vi "Generate Sync Cmd Event.vi"(4 "Task ID":string, 5 "Wait (F)":bool, 6 "Timeout (ms)":u32, 7 "AdHoc Cmd (\"\")":string, 8 "error in (no error)":errorcluster, 9 "vData":variant, 10 "AsyncCmd":T1, 11 "DLP2 in":refnum<class "DLP2.lvclass">) -> (0 "error out":errorcluster, 2 "Return Value":variant, 3 "DLP2 out":refnum<class "DLP2.lvclass">)   [LabVIEW 2022 SP3, in "DLP2.lvclass"]
doc: "Developed by Kevin Thompson\nkevin@thompsonengineering.net\n\nCopyright 2018\nThompson Engineering, LLC"
uses:
  DLP2.lvclass
  DataTypes/AsynCmd_Temp01--enum.ctl
  Common/Controls/TD Sync API Event Data.ctl
  Common/Controls/APIReturnCluster--Cluster.ctl
  Common/Controls/TD Sync API Task State.ctl
  Common/Controls/TD Async CmdMsg EventData--cluster.ctl
  DLP2.lvclass/DLP2.ctl
  Accessors/Get PublicEvents.vi
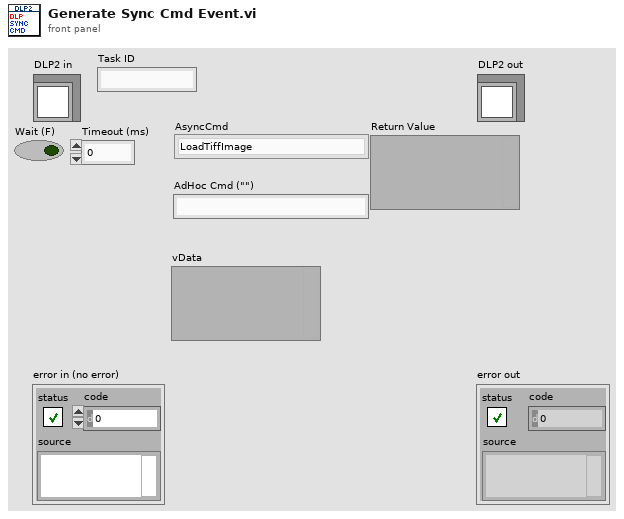
[diagram p1: front panel]
types:
  T1 = typedef "DLP2.lvclass/AsynCmd_Temp01--enum.ctl" = enum16{"LoadTiffImage"}
  T2 = typedef "TD Sync API Task State.ctl" = enum16{"Completed", "Executing", "Errored", "Pending"}
  T3 = typedef "TD Async CmdMsg EventData--cluster.ctl" = cluster{"Time Stamp":timestamp, "CmdMsg":string, "vData":variant}
  T4 = typedef "TD Sync API Event Data.ctl" = cluster{"Task":T5, "Command":variant, "Return Value":variant}
  T5 = typedef "APIReturnCluster--Cluster.ctl" = cluster{"Time Stamp":timestamp, "Timeout (ms)":u32, "Task State":T2, "Task Error":errorcluster, "Task ID":string, "Type":enum16{"API", "CMD"}}
  T6 = typedef "DLP2.lvclass/Public Events--cluster.ctl" = cluster{"Temp01.AsyncCmd Event":refnum<user-event>, "Temp01.AsyncMsg Event":refnum<user-event>, "stop process":refnum<user-event>, "API Incoming Event":refnum<user-event>, "API Executed Event":refnum<user-event>, "API Return Event":refnum<user-event>}
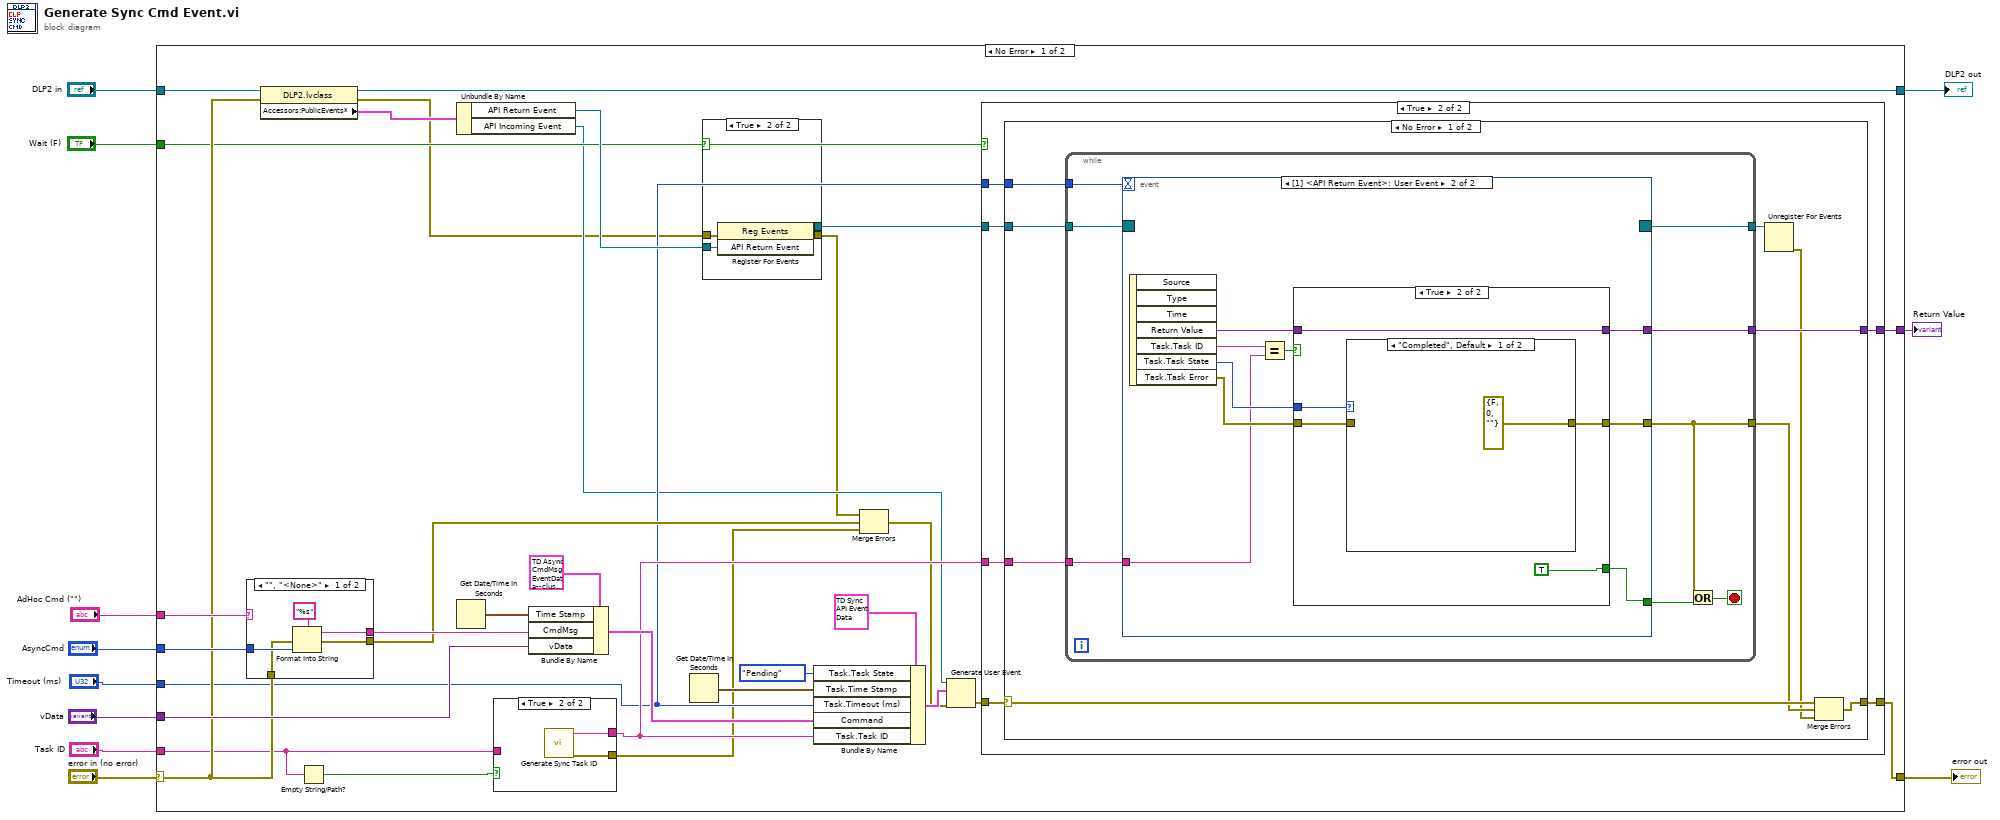
[diagram p0: block diagram]
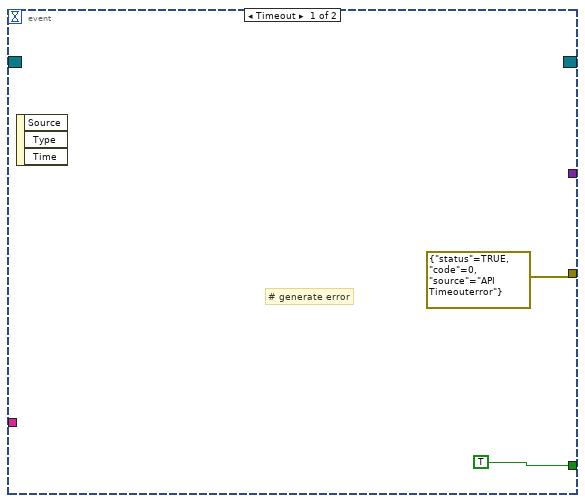
[diagram p3: hidden frame]
diagram:
  n1 = case shown="No Error" "error in (no error)" {
    selector: "error in (no error)" -> [w33 w102]
    tunnel: [w18 w102] -> w10
    tunnel: [w35 w101] -> w8
    tunnel: "DLP2 in" -> [w39 w101]
    tunnel: "AsyncCmd" -> [w37 _]
    tunnel: "vData" -> [w40 _]
    tunnel: "AdHoc Cmd (\"\")" -> [w36 _]
    tunnel: "Wait (F)" -> [w19 _]
    tunnel: "Task ID" -> [w28 _]
    tunnel: "Timeout (ms)" -> [w21 _]
    tunnel: [w17 _] -> w1
    frame No Error {
      n2 = case shown="\"\", \"<None>\"" w36 {
        selector: w36 -> [_ w99]
        tunnel: w37 -> [w97 _]
        tunnel: [w96 w99] -> w41
        tunnel: w33 -> [w95 w100]
        tunnel: [w94 w100] -> w38
        frame "", "<None>" {
          n3 = Format Into String(format string="%s", error in=w95, w97) -> (resulting string=w96:string, error out=w94:errorcluster)  [unwired: 1 in]
        }
        frame Default {
        }
      }
      n4 = property class="DLP2.lvclass"(reference=w39, error in=w33) -> (reference out=w35:refnum<class "DLP2.lvclass">, error out=w13:errorcluster, "Accessors:PublicEvents*"=w34:T6)
      n5 = Empty String/Path?(string/path=w28) -> (empty?=w27:bool)
      n6 = Unbundle By Name(w34) -> ("API Return Event"=w32:refnum<user-event>, "API Incoming Event"=w15:refnum<user-event>)
      n7 = Get Date/Time In Seconds() -> (seconds since 1Jan1904=w42:timestamp)
      n8 = case shown="True" w27 {
        tunnel: w28 -> [w86 _]
        tunnel: [w86 w88] -> w23
        tunnel: [_ w87] -> w14
        frame False {
        }
        frame True {
          n9 = call "Generate Sync Task ID.vi"() -> ("error out"=w87:errorcluster, "Task ID"=w88:string)  [unwired: 10 in]
        }
      }
      n10 = Bundle By Name(cluster=T3 {"Time Stamp"=timestamp(0 s since 1904-01-01), "CmdMsg"="", "vData"=variant} ("Async EvData"), "Time Stamp"=w42, "CmdMsg"=w41, "vData"=w40) -> (w24:T3)
      n11 = Get Date/Time In Seconds() -> (seconds since 1Jan1904=w25:timestamp)
      n12 = case shown="True" w19 {
        tunnel: w32 -> [_ w93]
        tunnel: [_ w92] -> w22
        tunnel: w13 -> [w89 w91]
        tunnel: [w89 w90] -> w12
        frame False {
        }
        frame True {
          n13 = register-events(error in=w91, w93) -> (reference out=w92:refnum<event-registration>, error out=w90:errorcluster)  [unwired: 1 in]
        }
      }
      n14 = Bundle By Name(cluster=T4 {"Task"={"Time Stamp"=timestamp(0 s since 1904-01-01), "Timeout (ms)"=0, "Task State"=enum."Completed", "Task Error"={"status"=FALSE, "code"=0, "source"=""}, "Task ID"="", "Type"=enum."API"}, "Command"=variant, "Return Value"=variant} ("API Event Data"), "Task.Task State"=TD_Sync_API_Task_State."Pending", "Task.Time Stamp"=w25, "Task.Timeout (ms)"=w21, "Command"=w24, "Task.Task ID"=w23) -> (w31:T4)
      n15 = Merge Errors(w12, w38, w14) -> (w16:errorcluster)
      n16 = Generate User Event(user event=w15, event data cluster=w31, error in=w16) -> (error out=w20:errorcluster)  [unwired: 1 in, 1 out]
      n17 = case shown="True" w19 {
        tunnel: w20 -> [w43 w49]
        tunnel: w21 -> [_ w48]
        tunnel: w22 -> [_ w47]
        tunnel: [_ w46] -> w17
        tunnel: [w43 w45] -> w18
        tunnel: w23 -> [_ w44]
        frame False {
        }
        frame True {
          n18 = case shown="No Error" w49 {
            selector: w49 -> [w54 w85]
            tunnel: w48 -> [w58 _]
            tunnel: w47 -> [w57 _]
            tunnel: [w56 _] -> w46
            tunnel: [w51 w85] -> w45
            tunnel: w44 -> [w50 _]
            frame No Error {
              n19 = while {
                tunnel: w58 -> [w59]
                tunnel: w57 -> [w66]
                tunnel: [w65] -> w56
                tunnel: [w63] -> w55
                tunnel: [w62] -> w53
                tunnel: w50 -> [w61]
                stop <- w64 stop-if-true
                n20 = event shown="[1] <API Return Event>: User Event" {
                  selector: w66 -> [_ _]
                  dyn-events: [_ _] -> w63
                  timeout: w59 -> [_ _]
                  tunnel: [_ w72] -> w65
                  tunnel: [errorcluster {"status"=TRUE, "code"=0, "source"="API Timeouterror"} ("Task Error") w71] -> w62
                  tunnel: [TRUE w69] -> w60
                  tunnel: w61 -> [_ w70]
                  event Timeout {
                    # "# generate error"
                    n21 = event-data() -> ()  [unwired: 1 in, 3 out]
                  }
                  event User Event {
                    n22 = event-data() -> ("Return Value"=w73:variant, "Task.Task ID"=w77:string, "Task.Task State"=w75:T2, "Task.Task Error"=w74:errorcluster)  [unwired: 1 in, 3 out]
                    n23 = Equal?(x=w77, y=w70) -> (x = y?=w76:bool)
                    n24 = case shown="True" w76 {
                      tunnel: w75 -> [_ w82]
                      tunnel: w74 -> [_ w81]
                      tunnel: [_ w80] -> w72
                      tunnel: w73 -> [_ w80]
                      tunnel: [_ w79] -> w71
                      tunnel: [_ TRUE] -> w69
                      frame False {
                      }
                      frame True {
                        n25 = case shown="\"Completed\", Default" w82 {
                          tunnel: w81 -> [_ w84]
                          tunnel: [errorcluster {"status"=FALSE, "code"=0, "source"=""} ("Task Error") w84] -> w79
                          frame "Completed", Default {
                          }
                          frame "Errored" {
                          }
                        }
                      }
                    }
                  }
                }
                n26 = Or(x=w62, y=w60) -> (x .or. y?=w64:bool)
              }
              n27 = Unregister For Events(event registration refnum=w55) -> (error out=w52:errorcluster)  [unwired: 1 in]
              n28 = Merge Errors(w54, w53, w52) -> (w51:errorcluster)
            }
            frame Error {
            }
          }
        }
      }
    }
    frame Error {
    }
  }
  "error out" <- w10
  "DLP2 out" <- w8
  "Return Value" <- w1
